vi "ReadRightShiftRegister.vi"(1 "reference":refnum<vi>) -> (0 "RightShiftRegister":T4)   [LabVIEW 2013]
uses:
  <vilib>/Utility/miscctls.llb/LVBoundsTypeDef.ctl
  <vilib>/Utility/miscctls.llb/LVPositionTypeDef.ctl
  <vilib>/Utility/miscctls.llb/LVRectTypeDef.ctl
panel:
  out "error out 17":errorcluster
  out "error out 16":errorcluster
  out "error out 15":errorcluster
  out "error out 14":errorcluster
  out "error out 13":errorcluster
  out "error out 12":errorcluster
  out "error out 11":errorcluster
  out "error out 10":errorcluster
  out "error out 9":errorcluster
  out "error out 8":errorcluster
  out "error out 7":errorcluster
  out "error out 6":errorcluster
  out "error out 5":errorcluster
  out "error out 4":errorcluster
  out "error out 3":errorcluster
  out "error out 2":errorcluster
  out "error out":errorcluster
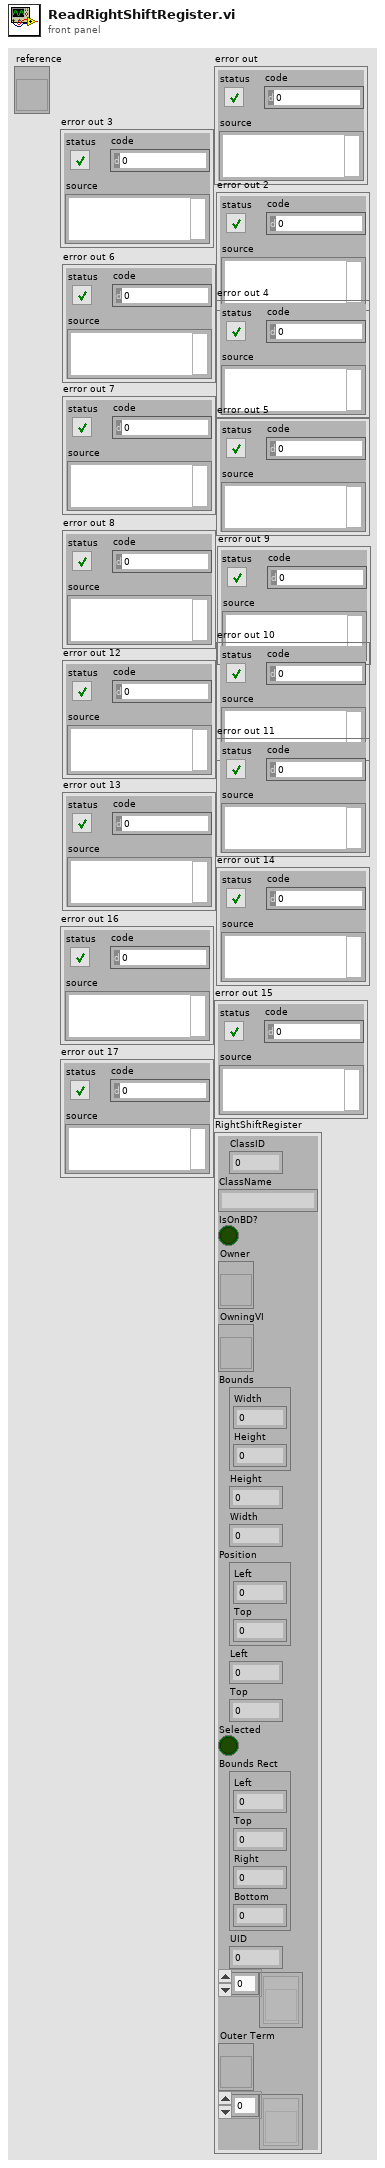
[diagram p1: front panel]
types:
  T1 = typedef "LVBoundsTypeDef.ctl" = cluster{"Width":u32, "Height":u32}
  T2 = typedef "LVPositionTypeDef.ctl" = cluster{"Left":i32, "Top":i32}
  T3 = typedef "LVRectTypeDef.ctl" = cluster{"Left":i16, "Top":i16, "Right":i16, "Bottom":i16}
  T4 = cluster{"ClassID":u32, "ClassName":string, "IsOnBD?":bool, "Owner":refnum<vi>, "OwningVI":refnum<vi>, "Bounds":T1, "Height":u32, "Width":u32, "Position":T2, "Left":i32, "Top":i32, "Selected":bool, "Bounds Rect":T3, "UID":i32, "InsideTerms[]":refnum<vi>[], "Outer Term":refnum<vi>, "LeftRegs[]":refnum<vi>[]}
  T5 = cluster{"ClassID":u32, "ClassName":string, "IsOnBD?":bool, "Owner":refnum<vi>, "OwningVI":refnum<vi>, "Bounds":T1, "Height":u32, "Width":u32, "Position":T2, "Left":i32, "Top":i32, "Selected":bool, "Bounds Rect":T3, "UID":i32, refnum<vi>[], "Outer Term":refnum<vi>, refnum<vi>[]}
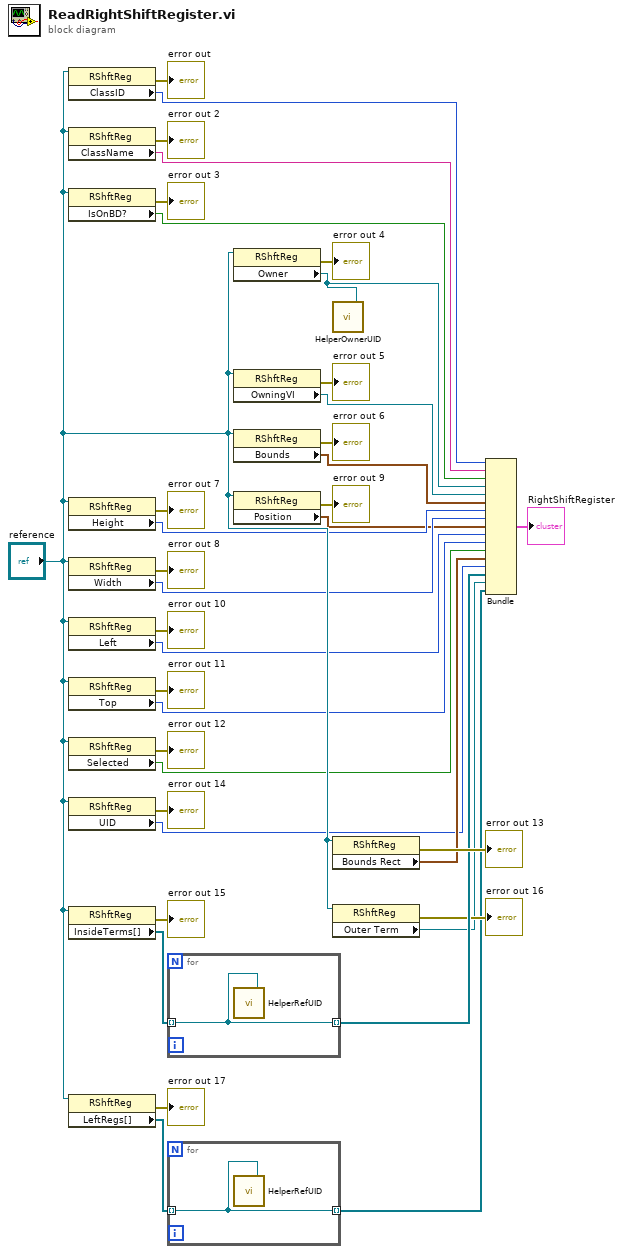
[diagram p0: block diagram]
diagram:
  n1 = property class="RShftReg"(reference="reference") -> (error out=→"error out":errorcluster, "ClassID"=w36:u32)  [unwired: 1 in, 1 out]
  n2 = property class="RShftReg"(reference="reference") -> (error out=→"error out 2":errorcluster, "ClassName"=w34:string)  [unwired: 1 in, 1 out]
  n3 = property class="RShftReg"(reference="reference") -> (error out=→"error out 3":errorcluster, "IsOnBD?"=w32:bool)  [unwired: 1 in, 1 out]
  n4 = property class="RShftReg"(reference="reference") -> (error out=→"error out 7":errorcluster, "Height"=w24:u32)  [unwired: 1 in, 1 out]
  n5 = property class="RShftReg"(reference="reference") -> (error out=→"error out 8":errorcluster, "Width"=w22:u32)  [unwired: 1 in, 1 out]
  n6 = property class="RShftReg"(reference="reference") -> (error out=→"error out 10":errorcluster, "Left"=w18:i32)  [unwired: 1 in, 1 out]
  n7 = property class="RShftReg"(reference="reference") -> (error out=→"error out 11":errorcluster, "Top"=w16:i32)  [unwired: 1 in, 1 out]
  n8 = property class="RShftReg"(reference="reference") -> (error out=→"error out 12":errorcluster, "Selected"=w14:bool)  [unwired: 1 in, 1 out]
  n9 = property class="RShftReg"(reference="reference") -> (error out=→"error out 14":errorcluster, "UID"=w10:i32)  [unwired: 1 in, 1 out]
  n10 = property class="RShftReg"(reference="reference") -> (error out=→"error out 15":errorcluster, "InsideTerms[]"=w8:refnum<vi>[])  [unwired: 1 in, 1 out]
  n11 = property class="RShftReg"(reference="reference") -> (error out=→"error out 17":errorcluster, "LeftRegs[]"=w3:refnum<vi>[])  [unwired: 1 in, 1 out]
  n12 = for {
    tunnel: w8 -> [w39] mode=indexing
    tunnel: [w39] -> w7 mode=indexing
    n13 = call "HelperRefUID.vi"("Text in"=w39) -> ()  [unwired: 1 out]
  }
  n14 = for {
    tunnel: w3 -> [w40] mode=indexing
    tunnel: [w40] -> w2 mode=indexing
    n15 = call "HelperRefUID.vi"("Text in"=w40) -> ()  [unwired: 1 out]
  }
  n16 = property class="RShftReg"(reference="reference") -> (error out=→"error out 4":errorcluster, "Owner"=w30:refnum<vi>)  [unwired: 1 in, 1 out]
  n17 = property class="RShftReg"(reference="reference") -> (error out=→"error out 5":errorcluster, "OwningVI"=w28:refnum<vi>)  [unwired: 1 in, 1 out]
  n18 = property class="RShftReg"(reference="reference") -> (error out=→"error out 6":errorcluster, "Bounds"=w26:T1)  [unwired: 1 in, 1 out]
  n19 = property class="RShftReg"(reference="reference") -> (error out=→"error out 9":errorcluster, "Position"=w20:T2)  [unwired: 1 in, 1 out]
  n20 = call "HelperOwnerUID.vi"("Generic in"=w30) -> ()  [unwired: 1 out]
  n21 = property class="RShftReg"(reference="reference") -> (error out=→"error out 13":errorcluster, "Bounds Rect"=w12:T3)  [unwired: 1 in, 1 out]
  n22 = property class="RShftReg"(reference="reference") -> (error out=→"error out 16":errorcluster, "Outer Term"=w5:refnum<vi>)  [unwired: 1 in, 1 out]
  n23 = Bundle("ClassID"=w36, "ClassName"=w34, "IsOnBD?"=w32, "Owner"=w30, "OwningVI"=w28, "Bounds"=w26, "Height"=w24, "Width"=w22, "Position"=w20, "Left"=w18, "Top"=w16, "Selected"=w14, "Bounds Rect"=w12, "UID"=w10, w7, "Outer Term"=w5, w2) -> (→"RightShiftRegister":T5)  [unwired: 1 in]
